vi "SR7270 Write and Read.vi"(8 "error in (no error)":errorcluster, 9 "Parameter(s)":string, 10 "Command Name":string, 11 "VISA resource name":refnum<visa-resource-name>) -> (0 "error out":errorcluster, 1 "Status":T1, 2 "Read":string, 3 "VISA resource name out":refnum<visa-resource-name>)   [LabVIEW 2016, in "SR7270 Drivers.lvclass"]
uses:
  SR7270 Drivers.lvclass
  <userlib>/_OpenG.lib/string/string.llb/Trim Whitespace (String)__ogtk.vi
panel:
  out "read < read?":bool
  out "time (ms)":u32
  # "Status Byte\n0 command complete\n1 invalid command\n2 command parameter error\n3 ref unlock\n4 output overload (read overload byte)\n5 new ADC values available\n6 input overload\n7 data available"
  # "Overload Byte\n0 X1\n1 Y1\n2 X2\n3 Y2\n4 CH1\n5 CH2\n6 CH3\n7 CH4"
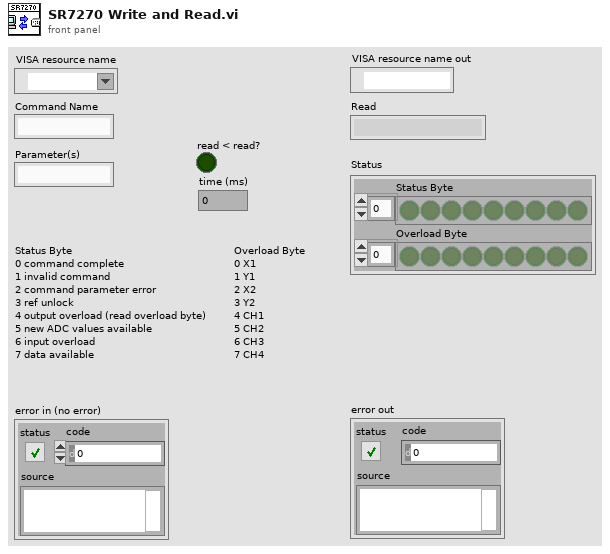
[diagram p1: front panel]
types:
  T1 = cluster{"Status Byte":bool[], "Overload Byte":bool[]}
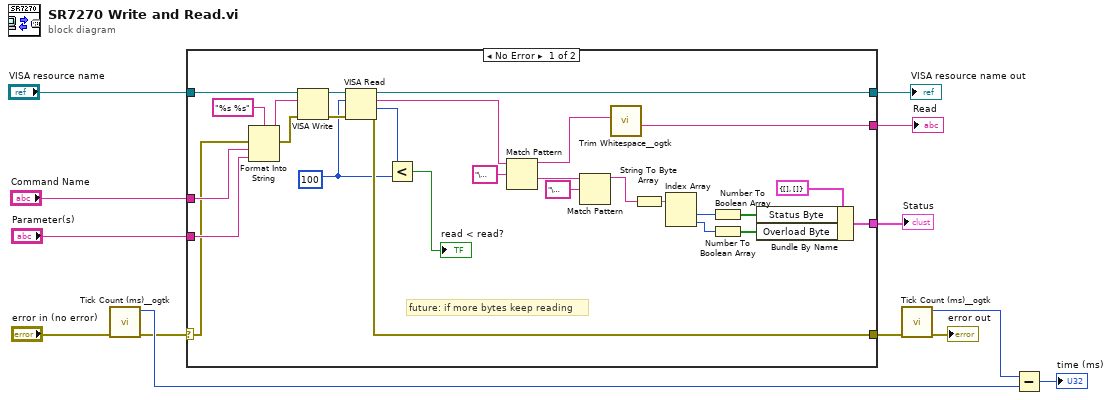
[diagram p0: block diagram]
diagram:
  n1 = call <userlib>:"Tick Count (ms)__ogtk.vi"("error in (no error)"="error in (no error)") -> ("error out"=w2:errorcluster, "millisecond timer value"=w5:u32)  [unwired: 9 in]
  n2 = case shown="No Error" w2 {
    selector: w2 -> [w19 w42]
    tunnel: "VISA resource name" -> [w41 w43]
    tunnel: [w33 _] -> w12
    tunnel: [w25 _] -> w11
    tunnel: "Command Name" -> [w23 _]
    tunnel: "Parameter(s)" -> [w22 _]
    tunnel: [w20 w42] -> w3
    tunnel: [w18 w43] -> w1
    frame No Error {
      w15 = u32 100 ("byte count")
      # "future: if more bytes keep reading"
      n3 = Format Into String(format string="%s %s" ("initial string"), error in=w19, w23, w22) -> (resulting string=w24:string, error out=w17:errorcluster)  [unwired: 1 in]
      n4 = VISA Write(VISA resource name=w41, write buffer=w24, error in (no error)=w17) -> (VISA resource name out=w40:refnum<visa-resource-name>, error out=w29:errorcluster)  [unwired: 1 out]
      n5 = VISA Read(VISA resource name=w40, byte count=w15, error in (no error)=w29) -> (VISA resource name out=w18:refnum<visa-resource-name>, read buffer=w36:string, return count=w16:u32, error out=w20:errorcluster)
      n6 = Less?(x=w16, y=w15) -> (x < y?=→"read < read?":bool)
      n7 = Match Pattern(string=w36, regular expression="\u0000") -> (before substring=w30:string, after substring=w34:string)  [unwired: 1 in, 2 out]
      n8 = Match Pattern(string=w34, regular expression="\u0000") -> (before substring=w32:string)  [unwired: 1 in, 3 out]
      n9 = call-poly <userlib>:"Trim Whitespace__ogtk.vi"("String in"=w30) -> ("String out"=w33:string)  [unwired: 6 in]
      n10 = String To Byte Array(string=w32) -> (unsigned byte array=w39:u8[])
      n11 = Index Array(array=w39) -> (element #1=w38:u8, element #2=w31:u8)  [unwired: 2 in]
      n12 = Number To Boolean Array(number=w38) -> (Boolean array=w27:bool[])
      n13 = Number To Boolean Array(number=w31) -> (Boolean array=w26:bool[])
      n14 = Bundle By Name(cluster=T1 {"Status Byte"=[], "Overload Byte"=[]} ("Status"), "Status Byte"=w27, "Overload Byte"=w26) -> (w25:T1)
    }
    frame Error {
    }
  }
  "Read" <- w12
  "Status" <- w11
  "VISA resource name out" <- w1
  n15 = call <userlib>:"Tick Count (ms)__ogtk.vi"("error in (no error)"=w3) -> ("error out"=→"error out":errorcluster, "millisecond timer value"=w6:u32)  [unwired: 9 in]
  n16 = Subtract(x=w6, y=w5) -> (x-y=→"time (ms)":u32)
